vi "parse connection string.vi"(11 "connection string in":string) -> (1 "service name":string, 2 "port":u16, 3 "address":string)   [LabVIEW 2015, in "TCP client.lvclass"]
uses:
  TCP client.lvclass
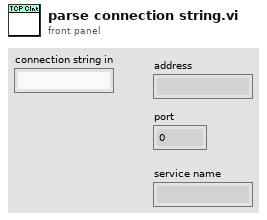
[diagram p1: front panel]
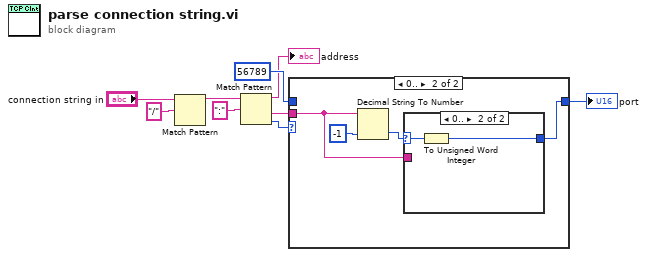
[diagram p0: block diagram]
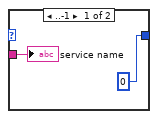
[diagram p3: hidden frame]
diagram:
  n1 = Match Pattern(string="connection string in", regular expression="/") -> (before substring=w8:string)  [unwired: 1 in, 3 out]
  n2 = Match Pattern(string=w8, regular expression=":") -> (before substring=→"address":string, after substring=w4:string, offset past match=w3:i32)  [unwired: 1 in, 1 out]
  n3 = case shown="0.." w3 {
    tunnel: w4 -> [_ w11]
    tunnel: [w10 w12] -> w5
    tunnel: u16 56789 ("port") -> [w10 _]
    frame ..-1 {
    }
    frame 0.. {
      n4 = Decimal String To Number(string=w11, default (0L)=-1 ("default (0 I32)")) -> (number=w13:i32)  [unwired: 1 in, 1 out]
      n5 = case shown="0.." w13 {
        selector: w13 -> [_ w18]
        tunnel: [u16 0 w17] -> w12
        tunnel: w11 -> [w16 _]
        frame ..-1 {
          "service name" <- w16
        }
        frame 0.. {
          n6 = To Unsigned Word Integer(number=w18) -> (unsigned 16bit integer=w17:u16)
        }
      }
    }
  }
  "port" <- w5
